vi "Find Red Pitayas VISA.vi"(6 "Timeout":i32=200, 7 "Logic tags":u16[](array[numeric])=[101, 102], 8 "Error In":errorcluster) -> (0 "Error Out":errorcluster, 1 "connections":refnum<visa-resource-name>[](array[refnum]), 2 "Device names":string[](array[string]), 5 "Logic tags out":u16[](array[numeric])=[101, 102])   [LabVIEW 2016, in "Red Pitaya Digitizer.lvclass"]
uses:
  Red Pitaya Digitizer.lvclass
  RP Core/RP Communicator VISA/RP Communicator VISA.lvclass
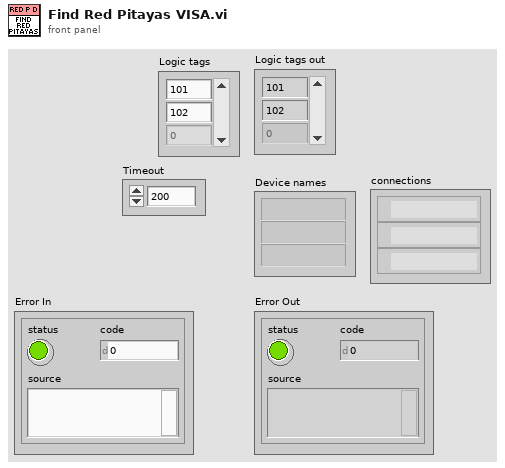
[diagram p1: front panel]
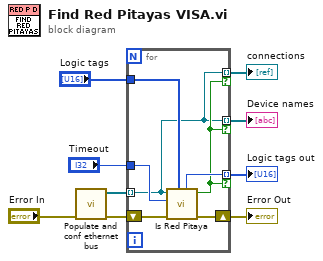
[diagram p0: block diagram]
diagram:
  n1 = call "Populate and conf ethernet bus.vi"("Error In"="Error In") -> ("Error Out"=w2:errorcluster, "Devices"=w1:refnum<visa-resource-name>[])  [unwired: 9 in]
  n2 = for {
    tunnel: "Timeout" -> [w11]
    tunnel: [w10] -> w8 mode=indexing if=w12
    shift-right: [w15] -> w6
    shift-left: w2 -> [w16]
    tunnel: [w10] -> w7 mode=indexing if=w12
    tunnel: "Logic tags" -> [w14]
    tunnel: [w13] -> w4 mode=indexing if=w12
    tunnel: w1 -> [w10] mode=indexing
    n3 = call "Is Red Pitaya.vi"("Logic tags"=w14, "Error In"=w16, "Timeout"=w11, "connection"=w10) -> ("Error Out"=w15:errorcluster, "Red Pitaya"=w12:bool, "Logic tag out"=w13:u16)  [unwired: 3 in, 2 out]
  }
  "Device names" <- w7
  "Error Out" <- w6
  "connections" <- w8
  "Logic tags out" <- w4
